vi "门禁开关监测界面.vi"() -> ()   [LabVIEW 2016, in "环境动力监测库.lvlib"]
panel:
  in  "智能门禁":bool
  out "x+1":u32
  in  "解除告警":bool
  out "告警内容":string
  out "X6-门禁开关_MJ":bool caption="状态"
  # "门禁开关监测"
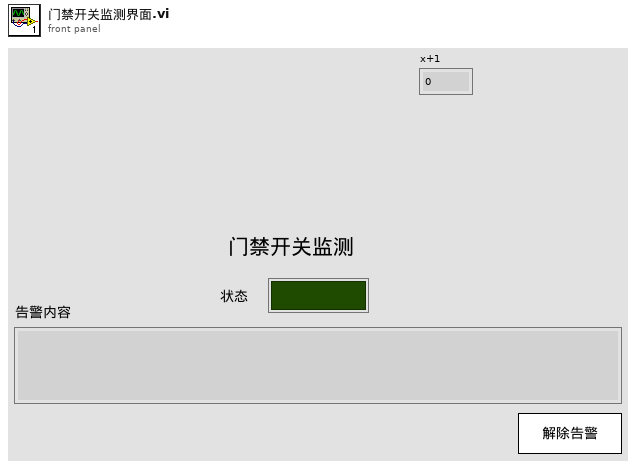
[diagram p1: front panel]
types:
  T1 = enum32{"Invalid", "Standard", "Closed", "Hidden", "Minimized", "Maximized"}
  T2 = cluster{"漏水监测输出":cluster{"漏水监测告警":bool, "告警内容":string}, "门禁监测输出":cluster{"门禁监测告警":bool, "告警内容":string}, "门禁监测输出2":cluster{"门禁监测告警":bool, "告警内容":string}, "温湿度监测输出":cluster{"温湿度监测告警":bool, "告警内容":string}, "烟雾监测输出":cluster{"烟雾监测告警":bool, "告警内容":string}, "空调监测输出":cluster{"空调监测告警":bool, "告警内容":string}, "自动重合闸输出":cluster{"自动重合闸告警":bool, "告警内容":string}, "红外入侵输出":cluster{"红外入侵告警":bool, "告警内容":string}, "振动输出":cluster{"振动告警":bool, "告警内容":string}, "UPS输出":cluster{"UPS告警":bool, "告警内容":string}, "蓄电池输出":cluster{"蓄电池告警":bool, "告警内容":string}, "蓄电池输出2":cluster{"蓄电池告警":bool, "告警内容":string}, "GPS输出":cluster{"定位告警":bool, "告警内容":string}, "北斗输出":cluster{"定位告警":bool, "告警内容":string}, "气象输出":cluster{"气象告警":bool, "告警内容":string}, "废液输出":cluster{"废液告警":bool, "告警内容":string}, "废液输出2":cluster{"废液告警":bool, "告警内容":string}}
  T3 = enum32{"Bad", "Idle", "Run top level", "Running"}
  T4 = cluster{"市电监测":bool, "用水量监测":bool, "烟雾监测":bool, "温度湿度":bool, "振动监测":bool, "红外入侵监测":bool, "漏水监测":bool, "门禁开关监测":bool, "门禁开关监测2":bool, "视频监测":bool, "UPS监测":bool, "空调监测":bool, "冰箱监测":bool, "排气扇监测":bool, "蓄电池监测":bool, "蓄电池监测2":bool, "GPS监测":bool, "北斗监测":bool, "气象监测":bool, "智能门禁监测":bool, "废液监测":bool, "废液监测2":bool}
  T5 = cluster{"漏水监测配置":cluster{"监测项描述:输出":string, "端口:":enum16{"AI0", "AI1", "AI2", "AI3", "AI4", "DI0", "DI1", "DI2", "DI3", "DI4", "DI5", "DI6", "DI7", "DO0", "DO1", "DO2", "DO3", "DO4", "DO5", "DO6", "DO7", "X0", "X1", "X2", "X3", "X4", "X5", "X6", "X7", "X8", "X9", "X10", "X11", "X12", "X13", "X14", "X15", "X16", "X17", "X18", "X19", "X20", "X21", "X22", "X23"}, "告警参数:":enum32{"禁用告警", "闭合告警", "断开告警"}, "传感器型号:":enum16{"PLC", "ZLAN", "ART"}, "声光告警启用":bool}, "门禁开关监测配置":cluster{"监测项描述:输出":string, "端口:":enum16{"AI0", "AI1", "AI2", "AI3", "AI4", "DI0", "DI1", "DI2", "DI3", "DI4", "DI5", "DI6", "DI7", "DO0", "DO1", "DO2", "DO3", "DO4", "DO5", "DO6", "DO7", "X0", "X1", "X2", "X3", "X4", "X5", "X6", "X7", "X8", "X9", "X10", "X11", "X12", "X13", "X14", "X15", "X16", "X17", "X18", "X19", "X20", "X21", "X22", "X23"}, "告警参数:":enum32{"禁用告警", "闭合告警", "断开告警"}, "传感器型号:":enum16{"PLC", "ZLAN", "ART"}, "声光告警启用":bool}, "门禁开关监测配置2":cluster{"监测项描述:输出":string, "端口:":enum16{"AI0", "AI1", "AI2", "AI3", "AI4", "DI0", "DI1", "DI2", "DI3", "DI4", "DI5", "DI6", "DI7", "DO0", "DO1", "DO2", "DO3", "DO4", "DO5", "DO6", "DO7", "X0", "X1", "X2", "X3", "X4", "X5", "X6", "X7", "X8", "X9", "X10", "X11", "X12", "X13", "X14", "X15", "X16", "X17", "X18", "X19", "X20", "X21", "X22", "X23"}, "告警参数:":enum32{"禁用告警", "闭合告警", "断开告警"}, "传感器型号:":enum16{"PLC", "ZLAN", "ART"}, "声光告警启用":bool}, "温湿度监测配置":cluster{"监测项描述:输出":string, "端口:":enum16{"AI0", "AI1", "AI2", "AI3", "AI4", "DI0", "DI1", "DI2", "DI3", "DI4", "DI5", "DI6", "DI7", "DO0", "DO1", "DO2", "DO3", "DO4", "DO5", "DO6", "DO7", "X0", "X1", "X2", "X3", "X4", "X5", "X6", "X7", "X8", "X9", "X10", "X11", "X12", "X13", "X14", "X15", "X16", "X17", "X18", "X19", "X20", "X21", "X22", "X23"}, "告警参数:":enum32{"禁用告警", "闭合告警", "断开告警"}, "传感器型号:":enum16{"PLC", "ZLAN", "ART"}, "声光告警启用":bool}, "烟雾监测配置":cluster{"监测项描述:输出":string, "端口:":enum16{"AI0", "AI1", "AI2", "AI3", "AI4", "DI0", "DI1", "DI2", "DI3", "DI4", "DI5", "DI6", "DI7", "DO0", "DO1", "DO2", "DO3", "DO4", "DO5", "DO6", "DO7", "X0", "X1", "X2", "X3", "X4", "X5", "X6", "X7", "X8", "X9", "X10", "X11", "X12", "X13", "X14", "X15", "X16", "X17", "X18", "X19", "X20", "X21", "X22", "X23"}, "告警参数:":enum32{"禁用告警", "闭合告警", "断开告警"}, "传感器型号:":enum16{"PLC", "ZLAN", "ART"}, "声光告警启用":bool}, "冰箱监测配置":cluster{"监测项描述:输出":string, "端口:":enum16{"AI0", "AI1", "AI2", "AI3", "AI4", "DI0", "DI1", "DI2", "DI3", "DI4", "DI5", "DI6", "DI7", "DO0", "DO1", "DO2", "DO3", "DO4", "DO5", "DO6", "DO7", "X0", "X1", "X2", "X3", "X4", "X5", "X6", "X7", "X8", "X9", "X10", "X11", "X12", "X13", "X14", "X15", "X16", "X17", "X18", "X19", "X20", "X21", "X22", "X23"}, "告警参数:":enum32{"禁用告警", "闭合告警", "断开告警"}, "传感器型号:":enum16{"PLC", "ZLAN", "ART"}, "声光告警启用":bool}, "排气扇监测配置":cluster{"监测项描述:输出":string, "端口:":enum16{"AI0", "AI1", "AI2", "AI3", "AI4", "DI0", "DI1", "DI2", "DI3", "DI4", "DI5", "DI6", "DI7", "DO0", "DO1", "DO2", "DO3", "DO4", "DO5", "DO6", "DO7", "X0", "X1", "X2", "X3", "X4", "X5", "X6", "X7", "X8", "X9", "X10", "X11", "X12", "X13", "X14", "X15", "X16", "X17", "X18", "X19", "X20", "X21", "X22", "X23"}, "告警参数:":enum32{"禁用告警", "闭合告警", "断开告警"}, "传感器型号:":enum16{"PLC", "ZLAN", "ART"}, "声光告警启用":bool}, "红外入侵监测配置":cluster{"监测项描述:输出":string, "端口:":enum16{"AI0", "AI1", "AI2", "AI3", "AI4", "DI0", "DI1", "DI2", "DI3", "DI4", "DI5", "DI6", "DI7", "DO0", "DO1", "DO2", "DO3", "DO4", "DO5", "DO6", "DO7", "X0", "X1", "X2", "X3", "X4", "X5", "X6", "X7", "X8", "X9", "X10", "X11", "X12", "X13", "X14", "X15", "X16", "X17", "X18", "X19", "X20", "X21", "X22", "X23"}, "告警参数:":enum32{"禁用告警", "闭合告警", "断开告警"}, "传感器型号:":enum16{"PLC", "ZLAN", "ART"}, "声光告警启用":bool}, "振动监测配置":cluster{"监测项描述:输出":string, "端口:":enum16{"AI0", "AI1", "AI2", "AI3", "AI4", "DI0", "DI1", "DI2", "DI3", "DI4", "DI5", "DI6", "DI7", "DO0", "DO1", "DO2", "DO3", "DO4", "DO5", "DO6", "DO7", "X0", "X1", "X2", "X3", "X4", "X5", "X6", "X7", "X8", "X9", "X10", "X11", "X12", "X13", "X14", "X15", "X16", "X17", "X18", "X19", "X20", "X21", "X22", "X23"}, "告警参数:":enum32{"禁用告警", "闭合告警", "断开告警"}, "传感器型号:":enum16{"PLC", "ZLAN", "ART"}, "声光告警启用":bool}, "废液监测配置":cluster{"监测项描述:输出":string, "端口:":enum16{"AI0", "AI1", "AI2", "AI3", "AI4", "DI0", "DI1", "DI2", "DI3", "DI4", "DI5", "DI6", "DI7", "DO0", "DO1", "DO2", "DO3", "DO4", "DO5", "DO6", "DO7", "X0", "X1", "X2", "X3", "X4", "X5", "X6", "X7", "X8", "X9", "X10", "X11", "X12", "X13", "X14", "X15", "X16", "X17", "X18", "X19", "X20", "X21", "X22", "X23"}, "告警参数:":enum32{"禁用告警", "闭合告警", "断开告警"}, "传感器型号:":enum16{"PLC", "ZLAN", "ART"}, "声光告警启用":bool}, "废液监测配置2":cluster{"监测项描述:输出":string, "端口:":enum16{"AI0", "AI1", "AI2", "AI3", "AI4", "DI0", "DI1", "DI2", "DI3", "DI4", "DI5", "DI6", "DI7", "DO0", "DO1", "DO2", "DO3", "DO4", "DO5", "DO6", "DO7", "X0", "X1", "X2", "X3", "X4", "X5", "X6", "X7", "X8", "X9", "X10", "X11", "X12", "X13", "X14", "X15", "X16", "X17", "X18", "X19", "X20", "X21", "X22", "X23"}, "告警参数:":enum32{"禁用告警", "闭合告警", "断开告警"}, "传感器型号:":enum16{"PLC", "ZLAN", "ART"}, "声光告警启用":bool}}
  T6 = cluster{"监测项描述:输出":string, "端口:":enum16{"AI0", "AI1", "AI2", "AI3", "AI4", "DI0", "DI1", "DI2", "DI3", "DI4", "DI5", "DI6", "DI7", "DO0", "DO1", "DO2", "DO3", "DO4", "DO5", "DO6", "DO7", "X0", "X1", "X2", "X3", "X4", "X5", "X6", "X7", "X8", "X9", "X10", "X11", "X12", "X13", "X14", "X15", "X16", "X17", "X18", "X19", "X20", "X21", "X22", "X23"}, "告警参数:":enum32{"禁用告警", "闭合告警", "断开告警"}, "传感器型号:":enum16{"PLC", "ZLAN", "ART"}, "声光告警启用":bool}
  T7 = enum16{"AI0", "AI1", "AI2", "AI3", "AI4", "DI0", "DI1", "DI2", "DI3", "DI4", "DI5", "DI6", "DI7", "DO0", "DO1", "DO2", "DO3", "DO4", "DO5", "DO6", "DO7", "X0", "X1", "X2", "X3", "X4", "X5", "X6", "X7", "X8", "X9", "X10", "X11", "X12", "X13", "X14", "X15", "X16", "X17", "X18", "X19", "X20", "X21", "X22", "X23"}
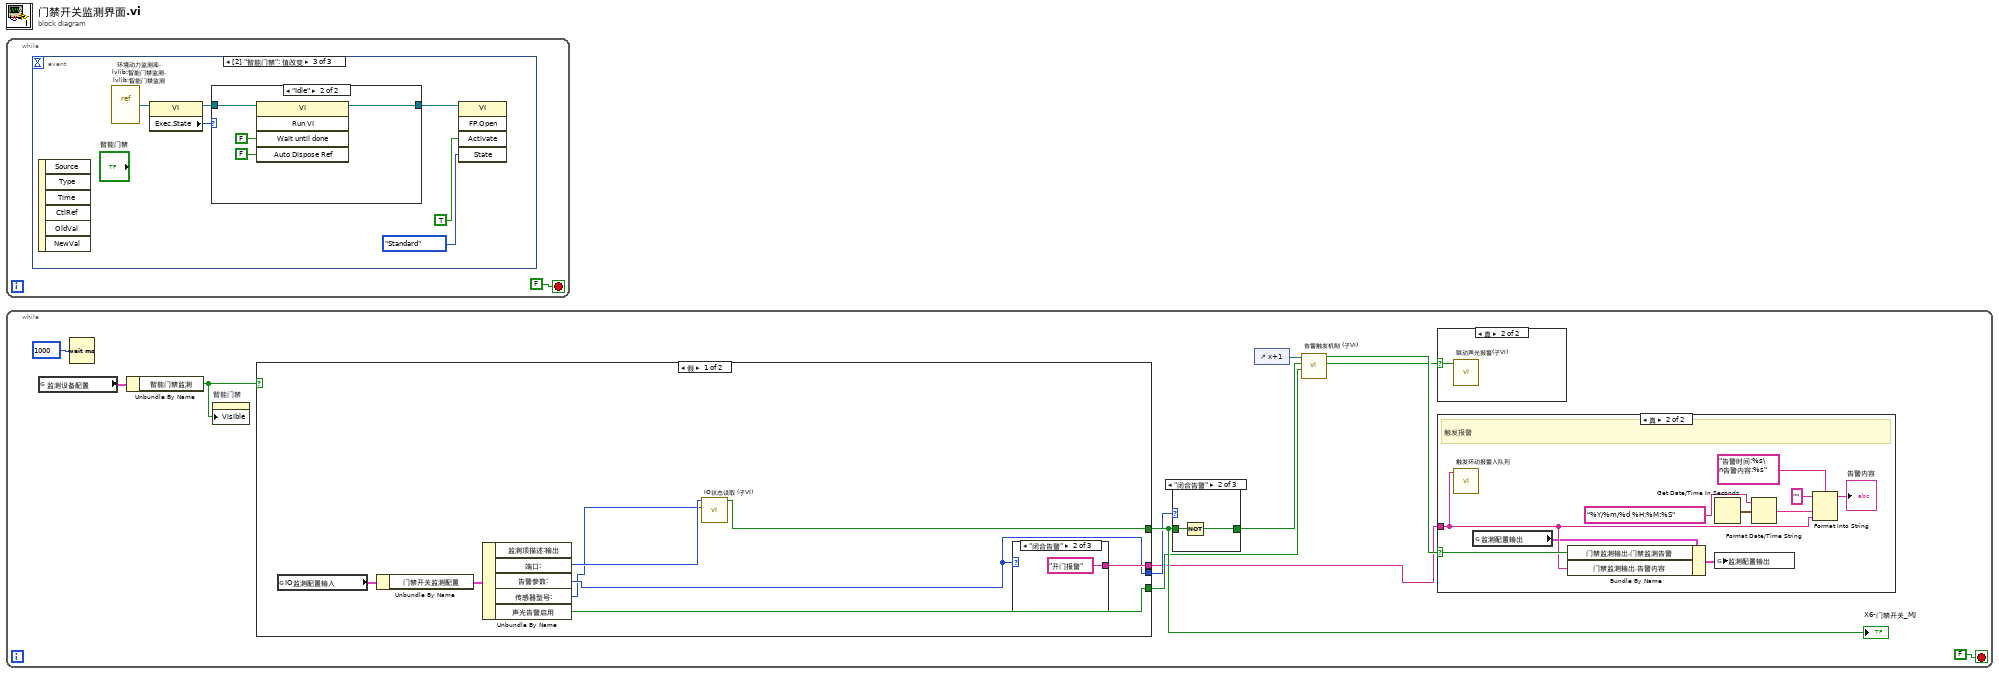
[diagram p0: block diagram]
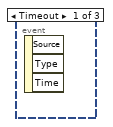
[diagram p2: hidden frame]
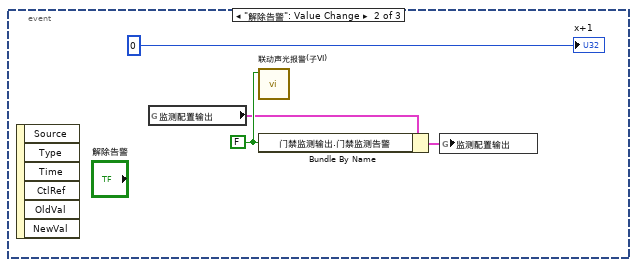
[diagram p3: hidden frame]
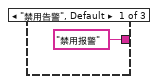
[diagram p5: hidden frame]
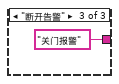
[diagram p6: hidden frame]
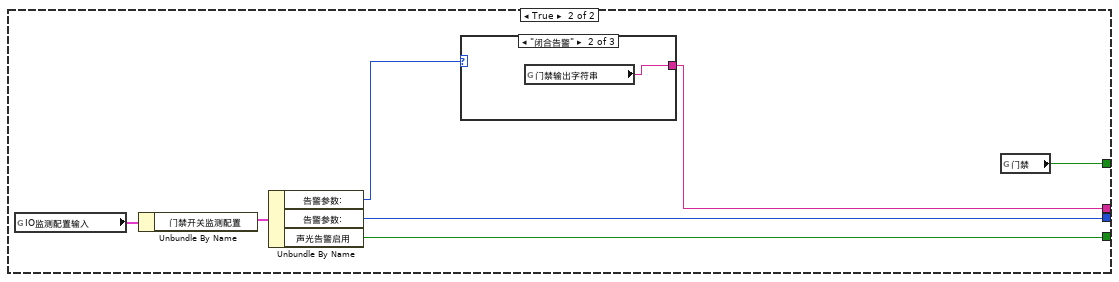
[diagram p7: hidden frame]
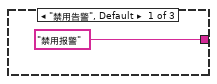
[diagram p8: hidden frame]
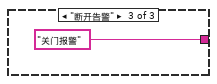
[diagram p9: hidden frame]
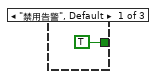
[diagram p12: hidden frame]
diagram:
  n1 = while {
    stop <- FALSE stop-if-true
    n2 = event shown="[2] \"智能门禁\": 值改变" {
      selector: _ -> [_ _ _]
      dyn-events: _ -> [_ _ _]
      timeout: _ -> [_ _ _]
      event Timeout {
        n3 = event-data() -> ()  [unwired: 1 in, 3 out]
      }
      event "解除告警": Value Change {
        w5 = FALSE
        n4 = event-data() -> ()  [unwired: 1 in, 6 out]
        n5 = global read "内部交互全局变量.vi" "监测配置输出"() -> (w3:T2)
        n6 = call "联动声光报警(子VI).vi"("布尔"=w5) -> ()  [unwired: 11 in]
        n7 = Bundle By Name(cluster=w3, "门禁监测输出.门禁监测告警"=w5) -> (w2:T2)
        n8 = global write "内部交互全局变量.vi" "监测配置输出"(w2) -> ()
        "x+1" <- u32 0 ("x+1")
      }
      event "智能门禁": Value Change {
        n9 = event-data() -> ()  [unwired: 1 in, 6 out]
        n10 = vi-ref "环境动力监测库.lvlib:智能门禁监测.lvlib:智能门禁监测.vi"() -> (w6:refnum<vi>)
        n11 = property class="VI"(reference=w6) -> (reference out=w10:refnum<vi>, "Exec.State"=w11:T3)  [unwired: 1 in, 1 out]
        n12 = case shown="\"Idle\"" w11 {
          tunnel: w10 -> [w12 w14]
          tunnel: [w12 w13] -> w7
          frame "Bad", Default {
          }
          frame "Idle" {
            n13 = invoke class="VI" method="Run VI"(reference=w14, "Wait until done"=FALSE ("结束前等待"), "Auto Dispose Ref"=FALSE ("自动销毁引用")) -> (reference out=w13:refnum<vi>)  [unwired: 2 in, 4 out]
          }
        }
        n14 = invoke class="VI" method="FP.Open"(reference=w7, "Activate"=TRUE ("激活？"), "State"=T1."Standard" ("状态")) -> ()  [unwired: 2 in, 5 out]
      }
    }
  }
  n15 = while {
    stop <- FALSE stop-if-true
    n16 = global read "断电保存全局变量.vi" "监测设备配置"() -> (w19:T4)
    n17 = Wait (ms)(milliseconds to wait=u32 1000 ("等待时间（毫秒）")) -> ()  [unwired: 1 out]
    n18 = Unbundle By Name(w19) -> ("智能门禁监测"=w18:bool)
    n19 = property on="智能门禁" class="Bool"("Visible"=w18) -> ()  [unwired: 2 in, 2 out]
    n20 = case shown="假" w18 {
      tunnel: [w29 w46] -> w26
      tunnel: [w32 w43] -> w25
      tunnel: [w34 w42] -> w22
      tunnel: [w33 w40] -> w17
      frame False {
        n21 = global read "断电保存全局变量.vi" "IO监测配置输入"() -> (w35:T5)
        n22 = Unbundle By Name(w35) -> ("门禁开关监测配置"=w36:T6)
        n23 = Unbundle By Name(w36) -> ("端口:"=w31:T7, "告警参数:"=w32:enum32{"禁用告警", "闭合告警", "断开告警"}, "传感器型号:"=w30:enum16{"PLC", "ZLAN", "ART"}, "声光告警启用"=w34:bool)  [unwired: 1 out]
        n24 = call "IO状态读取 (子VI).vi"("传感器型号:"=w30, "端口:"=w31) -> ("布尔"=w29:bool)  [unwired: 9 in]
        n25 = case shown="\"闭合告警\"" w32 {
          tunnel: ["禁用报警" ("日志信息") "开门报警" ("报警内容") "关门报警" ("日志信息")] -> w33
          frame "禁用告警", Default {
          }
          frame "闭合告警" {
          }
          frame "断开告警" {
          }
        }
      }
      frame True {
        n26 = global read "断电保存全局变量.vi" "IO监测配置输入"() -> (w44:T5)
        n27 = Unbundle By Name(w44) -> ("门禁开关监测配置"=w45:T6)
        n28 = Unbundle By Name(w45) -> ("告警参数:"=w41:enum32{"禁用告警", "闭合告警", "断开告警"}, "告警参数:"=w43:enum32{"禁用告警", "闭合告警", "断开告警"}, "声光告警启用"=w42:bool)
        n29 = case shown="\"闭合告警\"" w41 {
          tunnel: ["禁用报警" ("日志信息") w48 "关门报警" ("日志信息")] -> w40
          frame "禁用告警", Default {
          }
          frame "闭合告警" {
            n30 = global read "内部交互全局.vi" "门禁输出字符串"() -> (w48:string)
          }
          frame "断开告警" {
          }
        }
        n31 = global read "内部交互全局.vi" "门禁"() -> (w46:bool)
      }
    }
    "X6-门禁开关_MJ" <- w26
    n32 = case shown="\"闭合告警\"" w25 {
      tunnel: w26 -> [_ w63 w64]
      tunnel: [TRUE ("漏水监测输出") w62 w64] -> w23
      frame "禁用告警", Default {
      }
      frame "闭合告警" {
        n33 = Not(x=w63) -> (.not. x?=w62:bool)
      }
      frame "断开告警" {
      }
    }
    n34 = control-ref of="x+1"() -> (w24:refnum<vi>)
    n35 = call "告警触发机制 (子VI).vi"("声光告警启用"=w22, "状态输出"=w23, "Digital输入"=w24) -> ("声光告警"=w20:bool, "触发告警"=w21:bool)  [unwired: 7 in]
    n36 = case shown="真" w20 {
      selector: w20 -> [_ w50]
      frame False {
      }
      frame True {
        n37 = call "联动声光报警(子VI).vi"("布尔"=w50) -> ()  [unwired: 11 in]
      }
    }
    n38 = case shown="真" w21 {
      selector: w21 -> [_ w60]
      tunnel: w17 -> [_ w54]
      frame False {
      }
      frame True {
        # "触发报警"
        n39 = call "触发环动报警入队列.vi"("报警内容"=w54) -> ()  [unwired: 11 in]
        n40 = global read "内部交互全局变量.vi" "监测配置输出"() -> (w52:T2)
        n41 = Bundle By Name(cluster=w52, "门禁监测输出.门禁监测告警"=w60, "门禁监测输出.告警内容"=w54) -> (w51:T2)
        n42 = Get Date/Time In Seconds() -> (seconds since 1Jan1904=w57:timestamp)
        n43 = global write "内部交互全局变量.vi" "监测配置输出"(w51) -> ()
        n44 = Format Date/Time String(time format string (%c)="%Y/%m/%d %H:%M:%S" ("时间格式字符串(%c)"), seconds (now)=w57) -> (date/time string=w59:string)  [unwired: 1 in]
        n45 = Format Into String(format string="告警时间:%s\n告警内容:%s" ("格式字符串"), initial string="" ("初始字符串"), w59, w54) -> (resulting string=→"告警内容":string)  [unwired: 1 in, 1 out]
      }
    }
  }
